vi "Toggle Static PFI High or Low.vi"(0 "RFSG Handle In":refnum<k15>, 5 "Toggle Direction":i32(ring)=21001 items=["Digital Low"=21000, "Digital High"=21001], 11 "error in (no error)":errorcluster) -> (4 "RFSG Handle Out":refnum<k15>, 15 "error out":errorcluster {"code" format="%.0x"})   [LabVIEW 2018, in "SG.lvlib"]
uses:
  SG.lvlib
  <instrlib>/niRFSG/niRFSG.llb/niRFSG Signal Names.ctl
  <instrlib>/niRFSG/niRFSG.llb/niRFSG Signal Identifiers.ctl
  <instrlib>/niRFSG/niRFSG.llb/niRFSG Exported Signal Destinations.ctl
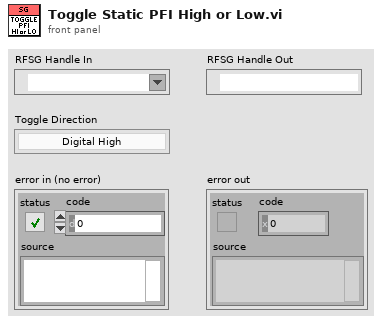
[diagram p1: front panel]
types:
  T1 = typedef "niRFSG Exported Signal Destinations.ctl" = string
  T2 = typedef "niRFSG Signal Identifiers.ctl" = string
  T3 = typedef "niRFSG Signal Names.ctl" = i32
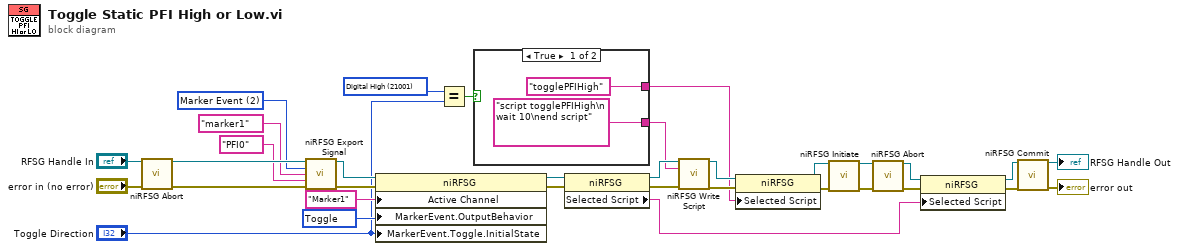
[diagram p0: block diagram]
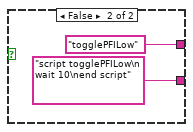
[diagram p2: hidden frame]
diagram:
  w1 = 21001 items=["Digital Low"=21000, "Digital High"=21001] ("Toggle Direction")
  w6 = T3 2 items=["Start Trigger", "Script Trigger", "Marker Event", "Ref Clock", "Started Event", "Done Event", "Configuration List Step Trigger", "Configuration Settled Event"] ("signal")
  w32 = 23001 items=["Pulse"=23000, "Toggle"=23001] ("Events:Marker:Output Behavior")
  n1 = call <instrlib>:"niRFSG Abort.vi"("instrument handle"="RFSG Handle In", "error in"="error in (no error)") -> ("instrument handle out"=w8:refnum<k15>, "error out"=w11:errorcluster)  [unwired: 12 in]
  n2 = call <instrlib>:"niRFSG Export Signal.vi"("instrument handle"=w8, "signal"=w6, "signal identifier"=T2 "marker1", "output terminal"=T1 "PFI0", "error in"=w11) -> ("instrument handle out"=w7:refnum<k15>, "error out"=w9:errorcluster)  [unwired: 9 in]
  n3 = property class="niRFSG"(reference=w7, error in=w9, "Active Channel"="Marker1", "MarkerEvent.OutputBehavior"=w32, "MarkerEvent.Toggle.InitialState"="Toggle Direction") -> (reference out=w31:refnum<k15>, error out=w30:errorcluster)
  n4 = Equal?(x=w1, y="Toggle Direction") -> (x = y?=w2:bool)
  n5 = case shown="True" w2 {
    tunnel: ["script togglePFIHigh\n   wait 10\nend script" ("script") "script togglePFILow\n   wait 10\nend script" ("script")] -> w25
    tunnel: ["togglePFIHigh" ("Arb:Selected Script") "togglePFILow" ("Arb:Selected Script")] -> w24
    frame True {
    }
    frame False {
    }
  }
  n6 = property class="niRFSG"(reference=w31, error in=w30) -> (reference out=w29:refnum<k15>, error out=w28:errorcluster, "Selected Script"=w21:string)
  n7 = call <instrlib>:"niRFSG Write Script.vi"("instrument handle"=w29, "script"=w25, "error in"=w28) -> ("instrument handle out"=w27:refnum<k15>, "error out"=w26:errorcluster)  [unwired: 11 in]
  n8 = property class="niRFSG"(reference=w27, error in=w26, "Selected Script"=w24) -> (reference out=w23:refnum<k15>, error out=w22:errorcluster)
  n9 = call <instrlib>:"niRFSG Initiate.vi"("instrument handle"=w23, "error in"=w22) -> ("instrument handle out"=w20:refnum<k15>, "error out"=w19:errorcluster)  [unwired: 12 in]
  n10 = call <instrlib>:"niRFSG Abort.vi"("instrument handle"=w20, "error in"=w19) -> ("instrument handle out"=w18:refnum<k15>, "error out"=w17:errorcluster)  [unwired: 12 in]
  n11 = property class="niRFSG"(reference=w18, error in=w17, "Selected Script"=w21) -> (reference out=w15:refnum<k15>, error out=w16:errorcluster)
  n12 = call <instrlib>:"niRFSG Commit.vi"("instrument handle"=w15, "error in"=w16) -> ("instrument handle out"=→"RFSG Handle Out":refnum<k15>, "error out"=→"error out":errorcluster)  [unwired: 12 in]
